vi "AlliGator Load Piccolo hist .bin Data.vi"(4 "# Pixels Y":i32, 6 "# Pixels X":i32, 8 "error in (no error)":errorcluster, 9 "# TCSPC Bins":i32, 11 "path in":path) -> (0 "error out":errorcluster, 2 "Array":u16[][][](array[numeric]), 3 "path out":path)   [LabVIEW 2021, in "AlliGator Files.lvlib"]
doc: "Loads Piccolo binned data."
uses:
  AlliGator Files.lvlib
panel:
  # "see the AlliGator License on the block diagram (Ctrl+E or Window:Show Block Diagram)"
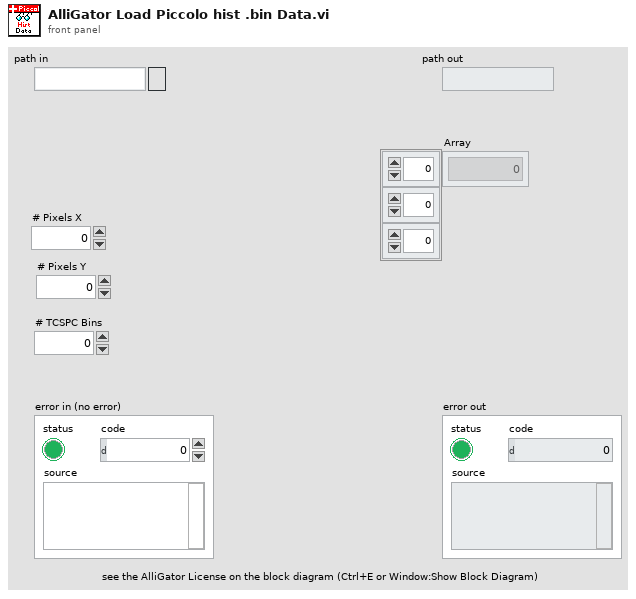
[diagram p1: front panel]
types:
  T1 = enum16{"big-endian, network order", "native, host order", "little-endian"}
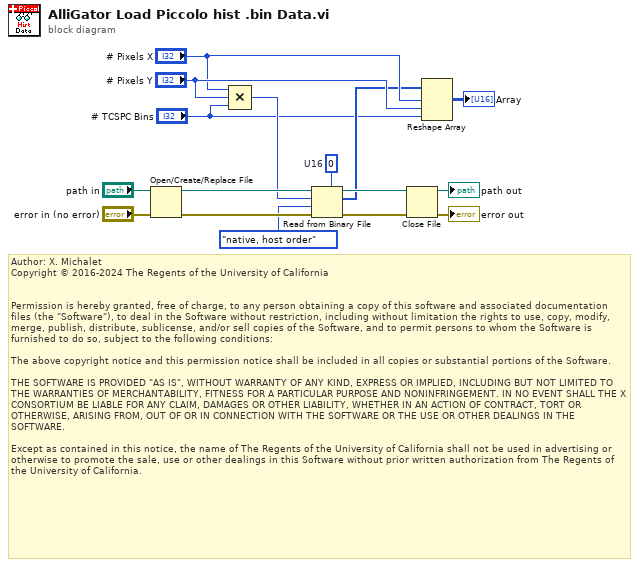
[diagram p0: block diagram]
diagram:
  w7 = u16 0  # U16
  # "Author: X. Michalet\nCopyright © 2016-2024 The Regents of the University of California\n \n\nPermission is hereby granted, free of charge, to any person obtaining a copy of this software and associated documentation files (the \"Software\"), to deal in the Software without restriction, including without limitation the rights to use, copy, modify, merge, publish, distribute, sublicense, and/or sell copies of the Software, and to permit persons to whom the Software is furnished to do so, subject to the following conditions:\n\nThe above copyright notice and this permission notice shall be included in all copies or substantial portions of the Software.\n\nTHE SOFTWARE IS PROVIDED \"AS IS\", WITHOUT WARRANTY OF ANY KIND, EXPRESS OR IMPLIED, INCLUDING BUT NOT LIMITED TO THE WARRANTIES OF MERCHANTABILITY, FITNESS FOR A PARTICULAR PURPOSE AND NONINFRINGEMENT. IN NO EVENT SHALL THE X CONSORTIUM BE LIABLE FOR ANY CLAIM, DAMAGES OR OTHER LIABILITY, WHETHER IN AN ACTION OF CONTRACT, TORT OR OTHERWISE, ARISING FROM, OUT OF OR IN CONNECTION WITH THE SOFTWARE OR THE USE OR OTHER DEALINGS IN THE SOFTWARE.\n\nExcept as contained in this notice, the name of The Regents of the University of California shall not be used in advertising or otherwise to promote the sale, use or other dealings in this Software without prior written authorization from The Regents of the University of California."
  n1 = Open/Create/Replace File(file path (use dialog)="path in", error in="error in (no error)") -> (refnum out=w13:refnum<file>, error out=w14:errorcluster)  [unwired: 4 in, 1 out]
  n2 = Compound Arithmetic op=MULTIPLY("# Pixels X", "# Pixels Y", "# TCSPC Bins") -> (w4:i32)
  n3 = Read from Binary File(5:w7, 8:w14, 9:T1."native, host order" ("byte order (0:big-endian, network order)"), 10:w4, 11:w13) -> (0:w2:errorcluster, 2:w5:u16[], 3:w15:refnum<file>)  [unwired: 1 in, 1 out]
  n4 = Close File(refnum=w15, error in=w2) -> (path=→"path out":path, error out=→"error out":errorcluster)
  n5 = Reshape Array(w5, "# Pixels X", "# Pixels Y", "# TCSPC Bins") -> (→"Array":u16[][][])
